vi "4.4.vi"() -> ()   [LabVIEW 2017]
panel:
  in  "数值":dbl
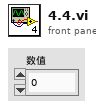
[diagram p1: front panel]
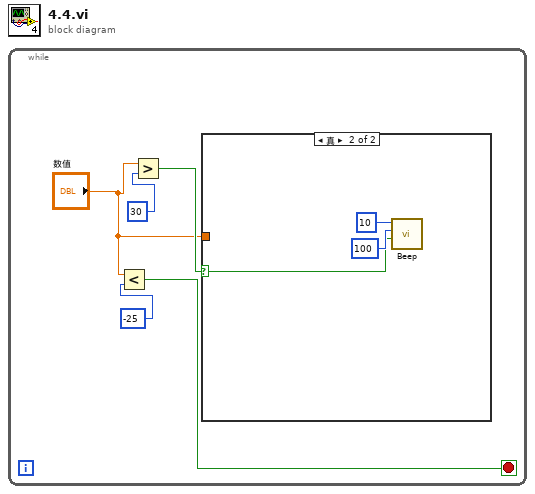
[diagram p0: block diagram]
diagram:
  n1 = while {
    stop <- w3 stop-if-true
    n2 = Less?(x="数值", y=-25) -> (x < y?=w3:bool)
    n3 = Greater?(x="数值", y=30) -> (0:w5:bool)
    n4 = case shown="真" w5 {
      selector: w5 -> [_ w6]
      tunnel: "数值" -> [_ _]
      frame False {
      }
      frame True {
        n5 = call <vilib>:"Beep.vi"("use system alert? (T)"=w6, "duration (msec)"=100, "frequency (Hz)"=10) -> ()  [unwired: 9 in]
      }
    }
  }
